vi "LTVUnicycleCtrl_Calculate.vi"(6 "RefAngularVelocity":dbl, 8 "RefLinearVelocity":dbl, 9 "RefPose":T2={"TRANSLATION"={"X"=0.0, "Y"=0.0}, "ROTATION"={"VALUE"=0.0, "COS"=1.0, "SIN"=0.0}} {"ROTATION"."SIN" format="%13.4f"; "ROTATION"."COS" format="%13.4f"; "ROTATION"."VALUE" format="%13.4f"; "TRANSLATION"."Y" format="%14.3f"; "TRANSLATION"."X" format="%14.3f"}, 10 "CurrentPose":T2={"TRANSLATION"={"X"=0.0, "Y"=0.0}, "ROTATION"={"VALUE"=0.0, "COS"=1.0, "SIN"=0.0}} {"ROTATION"."SIN" format="%13.4f"; "ROTATION"."COS" format="%13.4f"; "ROTATION"."VALUE" format="%13.4f"; "TRANSLATION"."Y" format="%14.3f"; "TRANSLATION"."X" format="%14.3f"}, 11 "in LTV_UNICYCLE_CONTROLLER":T5={"m_A"=[], "m_B"=[], "m_Q"=[], "m_R"=[], "States"=0, "Inputs"=0, "PoseError"={"TRANSLATION"={"X"=0.0, "Y"=0.0}, "ROTATION"={"VALUE"=0.0, "COS"=1.0, "SIN"=0.0}}, "PoseTolerance"={"TRANSLATION"={"X"=0.0, "Y"=0.0}, "ROTATION"={"VALUE"=0.0, "COS"=1.0, "SIN"=0.0}}, "Dt"=0.02, "Enabled"=FALSE} {"PoseTolerance"."ROTATION"."SIN" format="%13.4f"; "PoseTolerance"."ROTATION"."COS" format="%13.4f"; "PoseTolerance"."ROTATION"."VALUE" format="%13.4f"; "PoseTolerance"."TRANSLATION"."Y" format="%14.3f"; "PoseTolerance"."TRANSLATION"."X" format="%14.3f"; "PoseError"."ROTATION"."SIN" format="%13.4f"; "PoseError"."ROTATION"."COS" format="%13.4f"; "PoseError"."ROTATION"."VALUE" format="%13.4f"; "PoseError"."TRANSLATION"."Y" format="%14.3f"; "PoseError"."TRANSLATION"."X" format="%14.3f"}) -> (0 "Error":bool, 2 "ChassisSpeeds":T1 {"vOmega" format="%10.3f"; "vY" format="%10.3f"; "vX" format="%10.3f"}, 3 "out LTV_UNICYCLE_CONTROLLER":T5={"m_A"=[], "m_B"=[], "m_Q"=[], "m_R"=[], "States"=0, "Inputs"=0, "PoseError"={"TRANSLATION"={"X"=0.0, "Y"=0.0}, "ROTATION"={"VALUE"=0.0, "COS"=1.0, "SIN"=0.0}}, "PoseTolerance"={"TRANSLATION"={"X"=0.0, "Y"=0.0}, "ROTATION"={"VALUE"=0.0, "COS"=1.0, "SIN"=0.0}}, "Dt"=0.02, "Enabled"=FALSE} {"PoseTolerance"."ROTATION"."SIN" format="%13.4f"; "PoseTolerance"."ROTATION"."COS" format="%13.4f"; "PoseTolerance"."ROTATION"."VALUE" format="%13.4f"; "PoseTolerance"."TRANSLATION"."Y" format="%14.3f"; "PoseTolerance"."TRANSLATION"."X" format="%14.3f"; "PoseError"."ROTATION"."SIN" format="%13.4f"; "PoseError"."ROTATION"."COS" format="%13.4f"; "PoseError"."ROTATION"."VALUE" format="%13.4f"; "PoseError"."TRANSLATION"."Y" format="%14.3f"; "PoseError"."TRANSLATION"."X" format="%14.3f"})   [LabVIEW 2019, in "Trajectory_Library.lvlib"]
doc: "Create implicit model follower\n\nInputs:\n - A < states, states > -- Continuous system matrix of the plant being controlled.\n - B < states, inputs > -- Continuous input matrix of the plant being controlled.\n - A_Ref < states, states > -- Continuous system matrix whose dymanics should be followed.\n - B_Ref < states, inputs > -- Continuous input matrix x whose dymanics should be followed.\n\nOutputs:\n - Error -- If TRUE, an error occured."
uses:
  Trajectory_Library.lvlib
  LTV_UNICYCLE_CONTROLLER_STATE_ENUM.ctl
  <vilib>/Analysis/NI_AALBase.lvlib
  <vilib>/Analysis/baseanly.llb/Real A x B.vi
  <vilib>/Analysis/Matrix/Datatypes/RealMatrix.ctl
  <vilib>/Analysis/Matrix/NI_Matrix.lvlib
  LTV_UNICYCLE_CONTROLLER.ctl
  TRANSLATION2D.ctl
  ROTATION2D.ctl
  POSE2D.ctl
  CHASSIS_SPEEDS.ctl
panel:
  # "<States,States>"
  # "<States,Inputs>"
  # "<States, States>"
  # "<Inputs, Inputs>"
  # "<States,States>"
  # "<States,Inputs>"
  # "<States, States>"
  # "<Inputs, Inputs>"
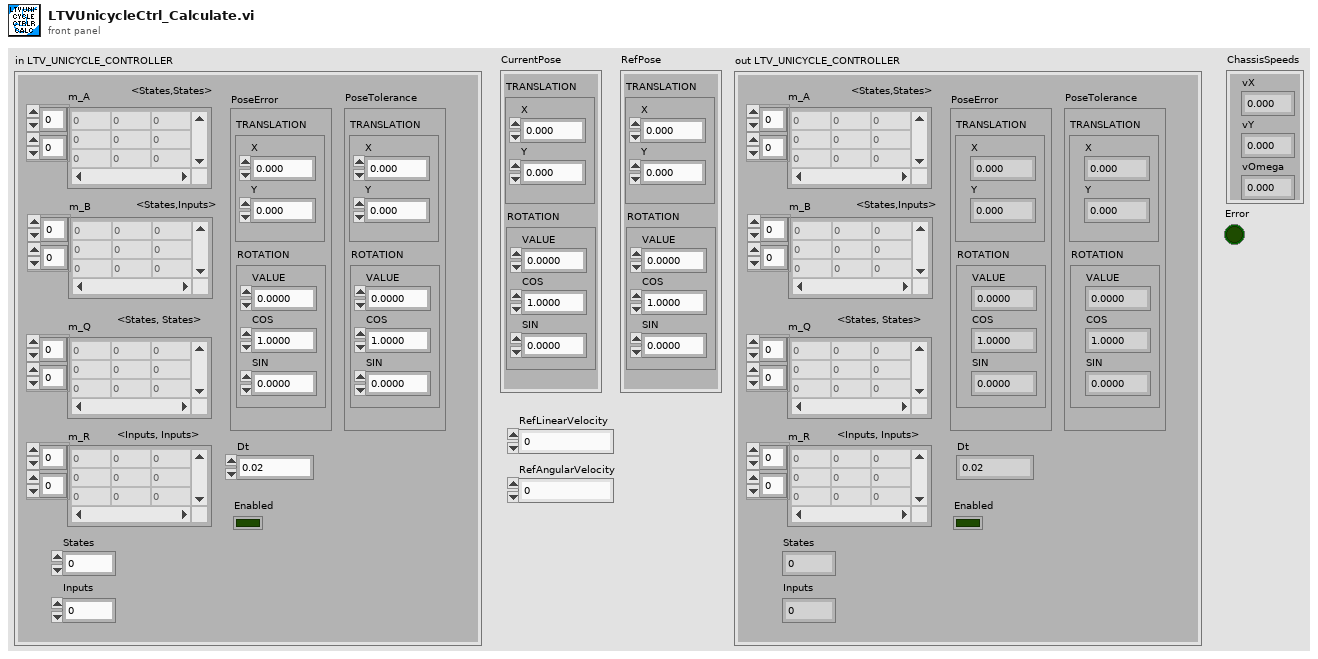
[diagram p1: front panel]
types:
  T1 = typedef "Trajectory_Library.lvlib/CHASSIS_SPEEDS.ctl" = cluster{"vX":dbl, "vY":dbl, "vOmega":dbl}
  T2 = typedef "Trajectory_Library.lvlib/POSE2D.ctl" = cluster{"TRANSLATION":T3, "ROTATION":T4}
  T3 = typedef "Trajectory_Library.lvlib/TRANSLATION2D.ctl" = cluster{"X":dbl, "Y":dbl}
  T4 = typedef "Trajectory_Library.lvlib/ROTATION2D.ctl" = cluster{"VALUE":dbl, "COS":dbl, "SIN":dbl}
  T5 = typedef "Trajectory_Library.lvlib/LTV_UNICYCLE_CONTROLLER.ctl" = cluster{"m_A":T6, "m_B":T6, "m_Q":T6, "m_R":T6, "States":i32, "Inputs":i32, "PoseError":T2, "PoseTolerance":T2, "Dt":dbl, "Enabled":bool}
  T6 = typedef "NI_Matrix.lvlib/RealMatrix.ctl" = dbl[][]
  T7 = typedef "Trajectory_Library.lvlib/LTV_UNICYCLE_CONTROLLER_STATE_ENUM.ctl" = enum16{"X", "Y", "HEADING"}
  T8 = typedef "Trajectory_Library.lvlib/LINEAR_QUADRATIC_REGULATOR.ctl" = cluster{"m_r":T6, "m_U":T6, "m_K":T6, "States":i32, "Inputs":i32}
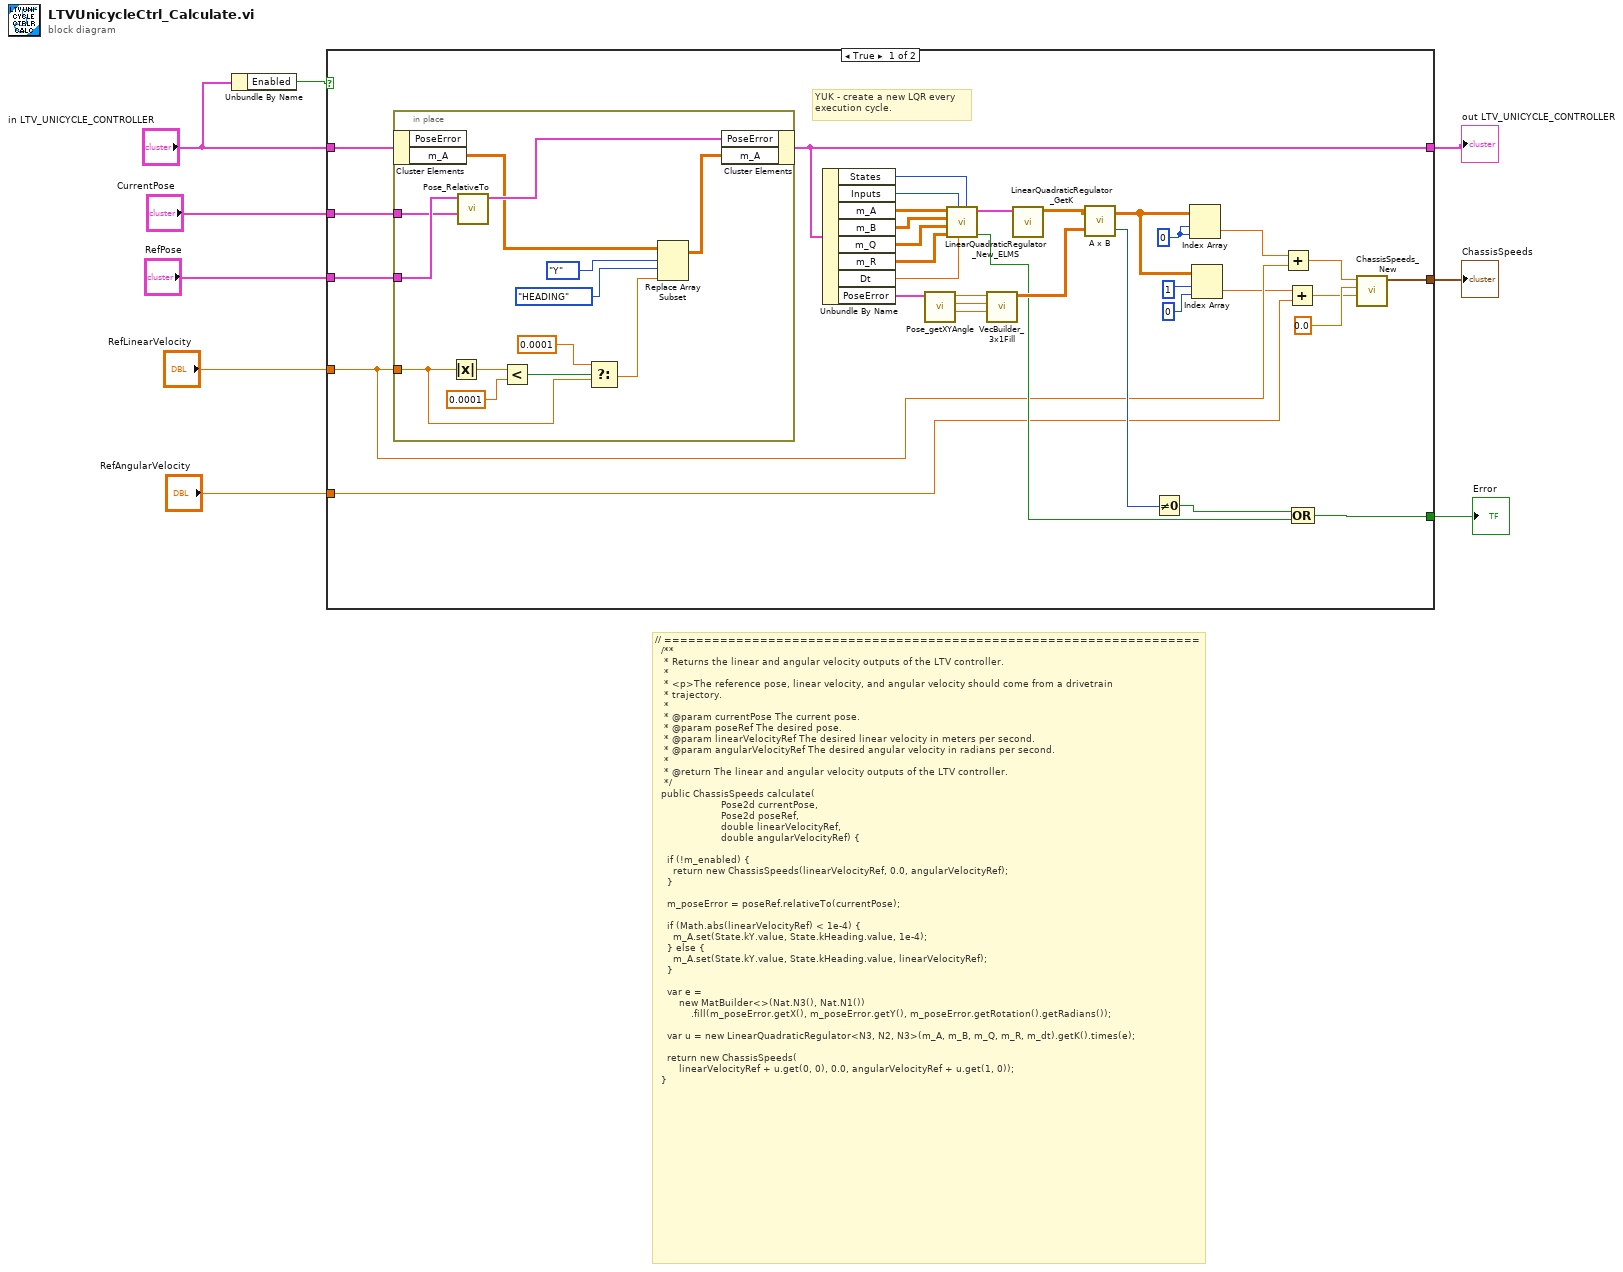
[diagram p0: block diagram]
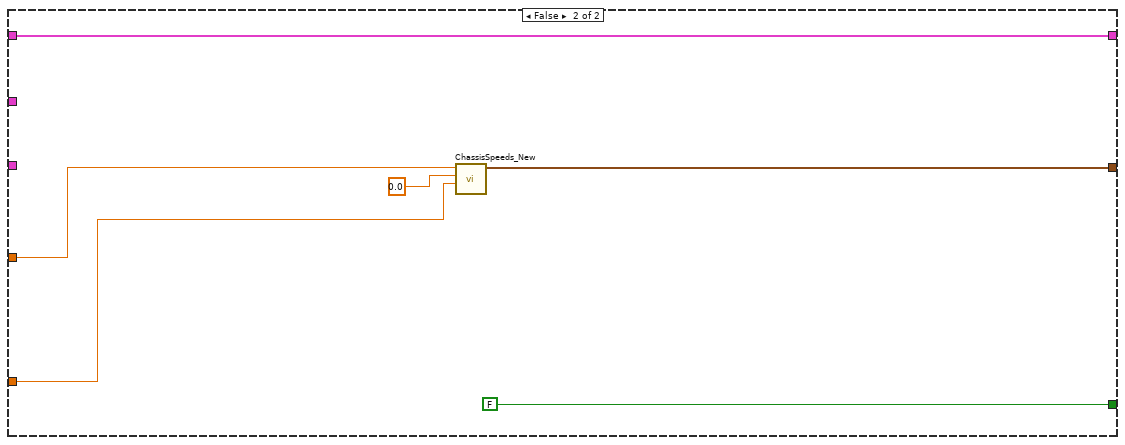
[diagram p2: hidden frame]
diagram:
  # "// ===================================================================\n  /**\n   * Returns the linear and angular velocity outputs of the LTV controller.\n   *\n   * <p>The reference pose, linear velocity, and angular velocity should come from a drivetrain\n   * trajectory.\n   *\n   * @param currentPose The current pose.\n   * @param poseRef The desired pose.\n   * @param linearVelocityRef The desired linear velocity in meters per second.\n   * @param angularVelocityRef The desired angular velocity in radians per second.\n   *\n   * @return The linear and angular velocity outputs of the LTV controller.\n   */\n  public ChassisSpeeds calculate(\n      \t               Pose2d currentPose, \n       \t              Pose2d poseRef, \n\t                     double linearVelocityRef, \n\t                     double angularVelocityRef) {\n\n    if (!m_enabled) {\n      return new ChassisSpeeds(linearVelocityRef, 0.0, angularVelocityRef);\n    }\n\n    m_poseError = poseRef.relativeTo(currentPose);\n\n    if (Math.abs(linearVelocityRef) < 1e-4) {\n      m_A.set(State.kY.value, State.kHeading.value, 1e-4);\n    } else {\n      m_A.set(State.kY.value, State.kHeading.value, linearVelocityRef);\n    }\n\n    var e =\n        new MatBuilder<>(Nat.N3(), Nat.N1())\n            .fill(m_poseError.getX(), m_poseError.getY(), m_poseError.getRotation().getRadians());\n\n    var u = new LinearQuadraticRegulator<N3, N2, N3>(m_A, m_B, m_Q, m_R, m_dt).getK().times(e);\n\n    return new ChassisSpeeds(\n        linearVelocityRef + u.get(0, 0), 0.0, angularVelocityRef + u.get(1, 0));\n  }"
  n1 = Unbundle By Name("in LTV_UNICYCLE_CONTROLLER") -> ("Enabled"=w9:bool)
  n2 = case shown="True" w9 {
    tunnel: "in LTV_UNICYCLE_CONTROLLER" -> [w43 w62]
    tunnel: [w40 w62] -> w7
    tunnel: [w10 FALSE] -> w6
    tunnel: [w22 w60] -> w5
    tunnel: "RefLinearVelocity" -> [w18 w59]
    tunnel: "RefAngularVelocity" -> [w17 w58]
    tunnel: "RefPose" -> [w42 _]
    tunnel: "CurrentPose" -> [w41 _]
    frame True {
      w16 = 0 ("index (row)")
      # "YUK - create a new LQR every\nexecution cycle."
      n3 = in-place {
        in-place-border: w42 -> [w56]
        in-place-border: w41 -> [w55]
        in-place-border: w18 -> [w45]
        n4 = in-place-cluster #1(w43) -> ("m_A"=w51:T6)  [unwired: 1 out]
        n5 = Absolute Value(x=w45) -> (abs(x)=w53:dbl)
        n6 = call "Pose_RelativeTo.vi"("other POSE"=w55, "in POSE"=w56) -> ("out POSE"=w54:T2)  [unwired: 9 in]
        n7 = Less?(x=w53, y=0.0001) -> (x < y?=w47:bool)
        n8 = Select(t=0.0001, s=w47, f=w45) -> (s? t:f=w44:dbl)
        n9 = Replace Array Subset(array=w51, new element=w44, index (row)=LTV_UNICYCLE_CONTROLLER_STATE_ENUM."Y" ("LTV_UNICYCLE_CONTROLLER_STATE"), index (col)=LTV_UNICYCLE_CONTROLLER_STATE_ENUM."HEADING" ("LTV_UNICYCLE_CONTROLLER_STATE")) -> (w50:T6)
        n10 = in-place-cluster #1("PoseError"=w54, "m_A"=w50) -> (w40:T5)
      }
      n11 = Unbundle By Name(w40) -> ("States"=w39:i32, "Inputs"=w38:i32, "m_A"=w37:T6, "m_B"=w36:T6, "m_Q"=w35:T6, "m_R"=w34:T6, "Dt"=w33:dbl, "PoseError"=w31:T2)
      n12 = call "Pose_getXYAngle.vi"("in POSE"=w31) -> ("Angle"=w28:dbl, "Y"=w29:dbl, "X"=w30:dbl)  [unwired: 8 in]
      n13 = call "LinearQuadraticRegulator_New_ELMS.vi"("States"=w39, "dt_Seconds"=w33, "Inputs"=w38, "Relms"=w34, "Qelms"=w35, "B"=w36, "A"=w37) -> ("Error"=w25:bool, "LinearQuadraticRegulator"=w32:T8)  [unwired: 3 in]
      n14 = call "VecBuilder_3x1Fill.vi"("R2"=w28, "R1"=w29, "R0"=w30) -> ("output matrix"=w26:T6)  [unwired: 8 in]
      n15 = call "LinearQuadraticRegulator_GetK.vi"("in LinearQuadraticRegulator"=w32) -> ("K"=w27:T6)  [unwired: 10 in]
      n16 = call-poly <vilib>:"A x B.vi"("B"=w26, "A"=w27) -> ("error"=w24:i32, "A x B"=w13:T6)
      n17 = Not Equal To 0?(x=w24) -> (x != 0?=w23:bool)
      n18 = Index Array(array=w13, index (row)=w16, index (col)=w16) -> (element=w12:dbl)
      n19 = Index Array(array=w13, index (row)=1, index (col)=0 ("index (row)")) -> (element=w11:dbl)
      n20 = Add(x=w12, y=w18) -> (x+y=w20:dbl)
      n21 = Add(x=w11, y=w17) -> (x+y=w19:dbl)
      n22 = Compound Arithmetic op=OR(w23, w25) -> (w10:bool)
      n23 = call "ChassisSpeeds_New.vi"("vAngular"=w19, "vY"=0.0, "vX"=w20) -> ("CHASSIS"=w22:T1)  [unwired: 8 in]
    }
    frame False {
      n24 = call "ChassisSpeeds_New.vi"("vAngular"=w58, "vY"=0.0, "vX"=w59) -> ("CHASSIS"=w60:T1)  [unwired: 8 in]
    }
  }
  "out LTV_UNICYCLE_CONTROLLER" <- w7
  "Error" <- w6
  "ChassisSpeeds" <- w5
